vi "Apply Corrections.vi"() -> ()   [LabVIEW 2011]
uses:
  <vilib>/Utility/file.llb/Read From Spreadsheet File (I64).vi
  <vilib>/Utility/file.llb/Read From Spreadsheet File (DBL).vi
panel:
  in  "LUT":i8[](array[numeric])=[0, 5, 10, 14, 18, 21, 23, 26, 28, 29, 31, 32, 33, 34, 35, 36, 36, 37, 38, 39, 40, 41, 42, 43, 43, 44, 45, 46, 46, 47, 48, 48, 49, 50, 50, 51, 52, 52, 53, 53, 54, 54, 55, 55, 56, 56, 57, 57, 58, 58, 59, 59, 60, 60, 61, 61, 62, 62, 63, 63, 64, 64, 65, 65, 65, 66, 66, 67, 67, 68, 68, 68, 69, 69, 70, 70, 70, 71, 71, 72, 72, 72, 73, 73, 74, 74, 74, 75, 75, 76, 76, 76, 77, 77, 78, 78, 78, 79, 79, 79, 80, 80, 81, 81, 81, 82, 82, 82, 83, 83, 83, 84, 84, 84, 85, 85, 85, 86, 86, 86, 87, 87, 87, 88, 88, 88, 89, 89, 89, 90, 90, 90, 91, 91, 91, 92, 92, 92, 93, 93, 93, 94, 94, 94, 95, 95, 95, 96, 96, 96, 97, 97, 97, 98, 98, 99, 99, 99, 100, 100, 101, 101, 101, 102, 102, 102, 103, 103, 103, 104, 104, 105, 105, 105, 106, 106, 106, 107, 107, 107, 108, 108, 109, 109, 109, 110, 110, 111, 111, 111, 112, 112, 113, 113, 113, 114, 114, 114, 115, 115, 116, 116, 117, 117, 117, 118, 118, 119, 119, 120, 120, 121, 121, 122, 122, 123, 123, 124, 124, 125, 125, 126, 127, 127, -128, -128, -127, -126, -126, -125, -124, -124, -123, -122, -122, -121, -120, -120, -119, -118, -117, -117, -116, -115, -115, -114, -113, -112, -112, -111, -110, -110, -109, -108, -107, -107]
  in  "Use\nregular\nLUT":bool
  in  "Load LUT":bool
  in  "DCborderWidth":i32=64
  in  "?":bool
  in  "?":bool
  in  "Use\nRestricted\nPhase\nChange":bool
  in  "stop":bool
  in  "Use \nPolynomial \nLUT":bool
  in  "Polynomial \nOrder":i32=7 min=3 max=7 step=1
  in  "Aberration \nCorrection":sgl[](array[numeric])=array[262144 elements]
  in  "Polynomial \nCoefficients":sgl[](array[numeric])=[128.0, 0.0, 0.0, 40.743664, 0.0, 0.0, 0.0, 0.0, 0.0, 0.0, 0.0, 0.0, 0.0, 0.0, 0.0, 0.0, 0.0, 0.0, 0.0, 0.0, 0.0, 0.0, 0.0, 0.0, 0.0, 0.0, 0.0, 0.0, 0.0, 0.0, 0.0, 0.0, 0.0, 0.0, 0.0, 0.0, 0.0, 0.0, 0.0, 0.0, 0.0, 0.0, 0.0, 0.0, 0.0, 0.0, 0.0, 0.0, 0.0, 0.0, 0.0, 0.0, 0.0, 0.0, 0.0, 0.0, 0.0, 0.0, 0.0, 0.0, 0.0, 0.0, 0.0, 0.0, 0.0, 0.0, 0.0, 0.0, 0.0, 0.0, 0.0, 0.0, 0.0, 0.0, 0.0, 0.0, 0.0, 0.0, 0.0, 0.0, 0.0, 0.0, 0.0, 0.0, 0.0, 0.0, 0.0, 0.0, 0.0, 0.0, 0.0, 0.0, 0.0, 0.0, 0.0, 0.0, 0.0, 0.0, 0.0, 0.0, 0.0, 0.0, 0.0, 0.0, 0.0, 0.0, 0.0, 0.0, 0.0, 0.0, 0.0, 0.0, 0.0, 0.0, 0.0, 0.0, 0.0, 0.0, 0.0, 0.0]
  in  "AlphaRPC":sgl=0.85
  in  "Compute\nAmplitudes":bool
  in  "Use\nAberration \nCorrection":bool
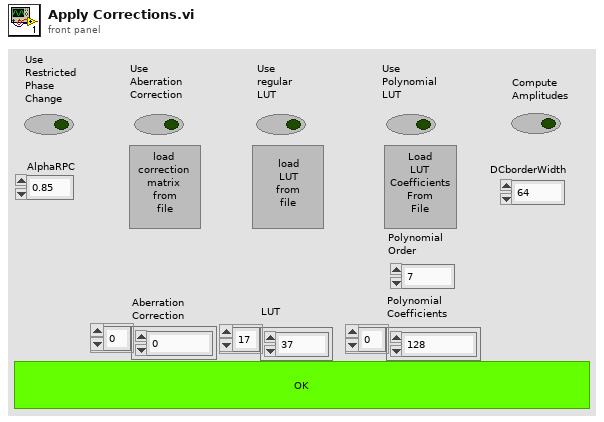
[diagram p1: front panel]
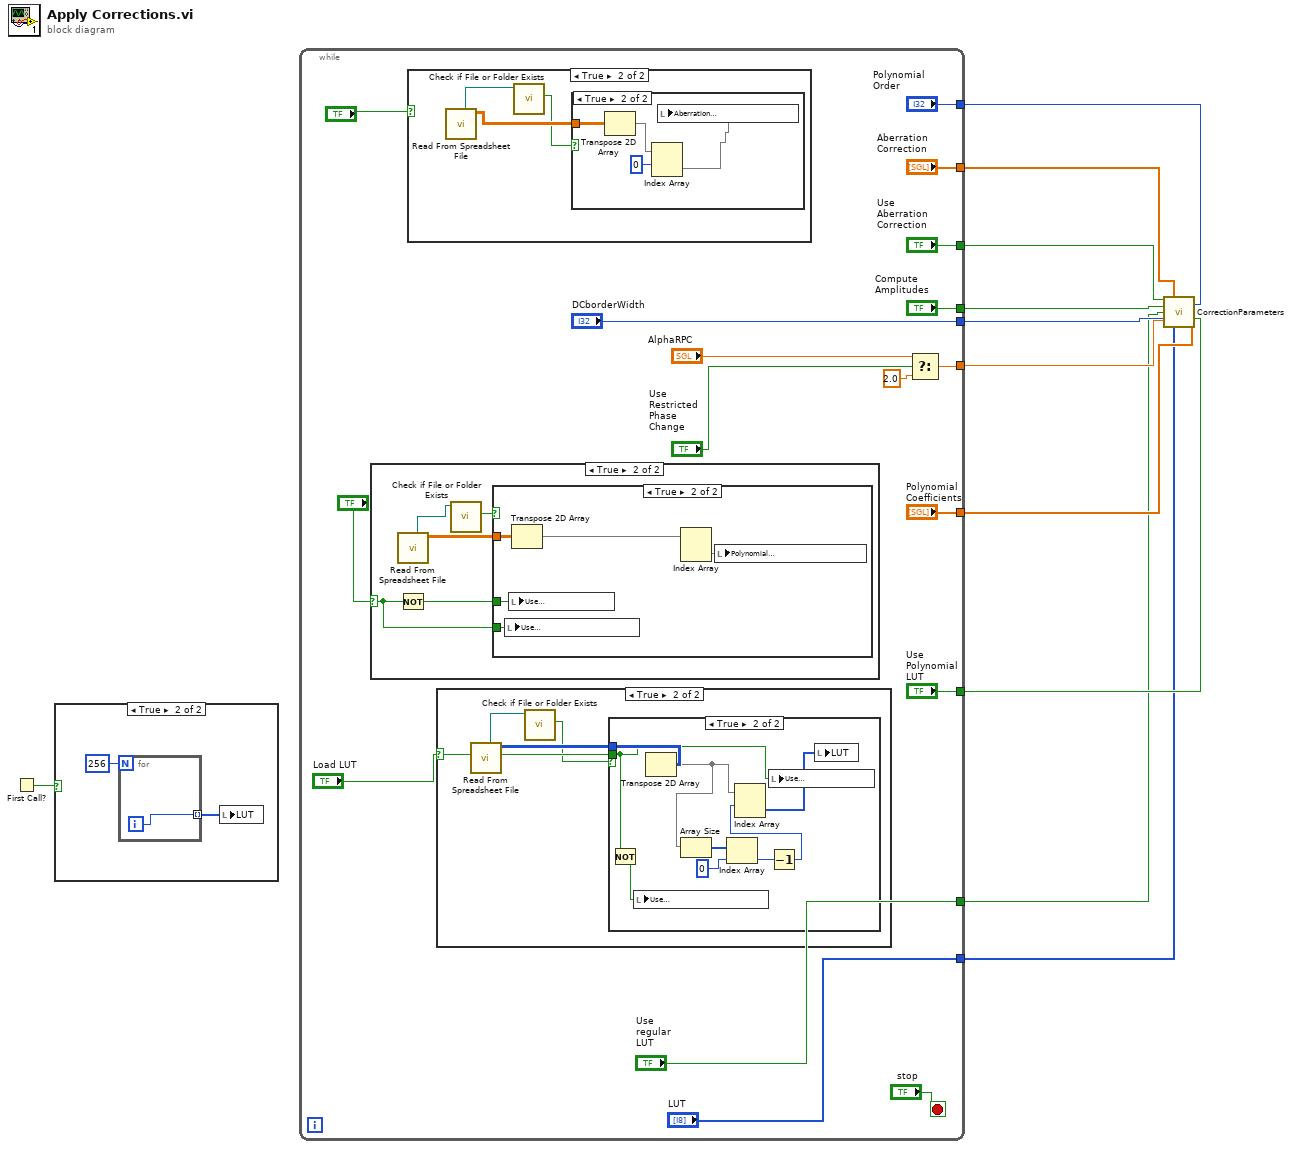
[diagram p0: block diagram]
diagram:
  n1 = First Call?() -> (First Call?: T/F=w1:bool)
  n2 = case shown="True" w1 {
    frame False {
    }
    frame True {
      n3 = for {
        N: 256 -> [_]
        tunnel: [w14] -> w12 mode=indexing
        i -> [w14]
      }
      n4 = local write "LUT"(w12) -> ()
    }
  }
  n5 = while {
    tunnel: ["Use\nAberration \nCorrection"] -> w11
    tunnel: ["Compute\nAmplitudes"] -> w10
    tunnel: [w21] -> w9
    tunnel: ["Polynomial \nCoefficients"] -> w8
    tunnel: ["Aberration \nCorrection"] -> w7
    tunnel: ["Polynomial \nOrder"] -> w6
    tunnel: ["Use \nPolynomial \nLUT"] -> w5
    tunnel: ["DCborderWidth"] -> w4
    tunnel: ["Use\nregular\nLUT"] -> w3
    tunnel: ["LUT"] -> w2
    stop <- "stop" stop-if-true
    n6 = case shown="True" "?" {
      selector: "?" -> [_ w52]
      frame False {
      }
      frame True {
        n7 = call-poly <vilib>:"Read From Spreadsheet File.vi"() -> ("all rows"=w56:dbl[][], "new file path (Not A Path if cancelled)"=w55:path)  [unwired: 7 in, 3 out]
        n8 = Not(x=w52) -> (.not. x?=w53:bool)
        n9 = call <vilib>:"Check if File or Folder Exists.vi"("path"=w55) -> ("file or folder exists?"=w54:bool)  [unwired: 8 in, 2 out]
        n10 = case shown="True" w54 {
          tunnel: w56 -> [_ w61]
          tunnel: w53 -> [_ w58]
          tunnel: w52 -> [_ w57]
          frame False {
          }
          frame True {
            n11 = local write "Use \nPolynomial \nLUT"(w57) -> ()
            n12 = local write "Use\nregular\nLUT"(w58) -> ()
            n13 = Transpose 2D Array(2D array=w61) -> (transposed array=w59:dbl[][])
            n14 = Index Array(array=w59) -> (element=w60:dbl[])  [unwired: 2 in]
            n15 = local write "Polynomial \nCoefficients"(w60) -> ()
          }
        }
      }
    }
    n16 = case shown="True" "?" {
      frame False {
      }
      frame True {
        n17 = call-poly <vilib>:"Read From Spreadsheet File.vi"() -> ("all rows"=w47:dbl[][], "new file path (Not A Path if cancelled)"=w46:path)  [unwired: 7 in, 3 out]
        n18 = call <vilib>:"Check if File or Folder Exists.vi"("path"=w46) -> ("file or folder exists?"=w45:bool)  [unwired: 8 in, 2 out]
        n19 = case shown="True" w45 {
          tunnel: w47 -> [_ w51]
          frame False {
          }
          frame True {
            n20 = Transpose 2D Array(2D array=w51) -> (transposed array=w50:dbl[][])
            n21 = Index Array(array=w50, index (row)=0) -> (element=w48:dbl[])  [unwired: 1 in]
            n22 = local write "Aberration \nCorrection"(w48) -> ()
          }
        }
      }
    }
    n23 = case shown="True" "Load LUT" {
      selector: "Load LUT" -> [_ w34]
      frame False {
      }
      frame True {
        n24 = call-poly <vilib>:"Read From Spreadsheet File.vi"() -> ("all rows"=w35:i64[][], "new file path (Not A Path if cancelled)"=w33:path)  [unwired: 7 in, 3 out]
        n25 = call <vilib>:"Check if File or Folder Exists.vi"("path"=w33) -> ("file or folder exists?"=w32:bool)  [unwired: 8 in, 2 out]
        n26 = case shown="True" w32 {
          tunnel: w35 -> [_ w44]
          tunnel: w34 -> [_ w37]
          frame False {
          }
          frame True {
            n27 = Not(x=w37) -> (.not. x?=w36:bool)
            n28 = local write "Use \nPolynomial \nLUT"(w36) -> ()
            n29 = Transpose 2D Array(2D array=w44) -> (transposed array=w40:i64[][])
            n30 = Array Size(array=w40) -> (size(s)=w39:i32[])
            n31 = Index Array(array=w39, index=0) -> (element=w41:i32)
            n32 = local write "Use\nregular\nLUT"(w37) -> ()
            n33 = Decrement(x=w41) -> (x-1=w38:i32)
            n34 = Index Array(array=w40, index (row)=w38) -> (element=w43:i64[])  [unwired: 1 in]
            n35 = local write "LUT"(w43) -> ()
          }
        }
      }
    }
    n36 = Select(t="AlphaRPC", s="Use\nRestricted\nPhase\nChange", f=sgl 2.0) -> (s? t:f=w21:sgl)
  }
  n37 = call "CorrectionParameters.vi"("Aberration Correction On"=w11, "Aberration Correction"=w7, "Polynomial Order"=w6, "SaveAmplitudes"=w10, "Polynomial Coefficients"=w8, "useLUT"=w3, "DCborderWidth"=w4, "Use polynomial LUT"=w5, "LUT"=w2, "AlphaRPC"=w9) -> ()  [unwired: 4 in, 2 out]
